vi "Get Category.vi"(8 "error in (no error)":errorcluster, 11 "RTResourceUtilitzation editor node in":refnum<class "RTResourceUtilitzation editor node.lvclass">) -> (0 "error out":errorcluster, 2 "Category":string, 3 "RTResourceUtilitzation editor node out":refnum<class "RTResourceUtilitzation editor node.lvclass">)   [LabVIEW 2014, in "RTResourceUtilitzation editor node.lvclass"]
uses:
  RTResourceUtilitzation editor node.lvclass
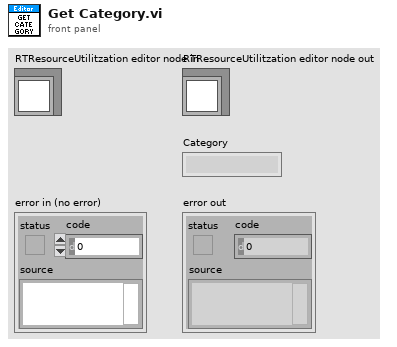
[diagram p1: front panel]
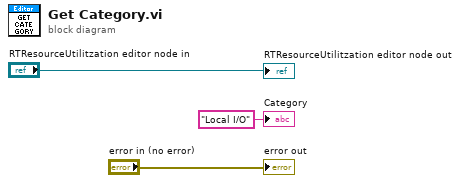
[diagram p0: block diagram]
diagram:
  "error out" <- "error in (no error)"
  "RTResourceUtilitzation editor node out" <- "RTResourceUtilitzation editor node in"
  "Category" <- "Local I/O" ("Category")
